vi "_UtilsRandomStringValue.vi"(1 "factor":dbl=100.0) -> (0 "random value":string)   [LabVIEW 2014, in "examples.lvlib"]
uses:
  examples.lvlib
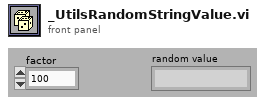
[diagram p1: front panel]
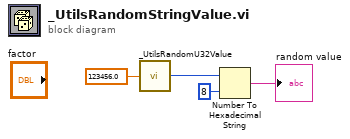
[diagram p0: block diagram]
diagram:
  n1 = call "_UtilsRandomU32Value.vi"("factor"=123456.0) -> ("random value"=w3:u32)
  n2 = Number To Hexadecimal String(1:i16 8 ("width (-)"), 2:w3) -> (0:→"random value":string)
